vi "Img Crop.vi"(8 "error in (no error)":errorcluster, 10 "Rectangle":T1, 11 "Image Src":T2) -> (0 "error out":errorcluster, 3 "Image Out":T2)   [LabVIEW 2018, in "Image Process.lvclass"]
uses:
  Image Process.lvclass
  <vilib>/vision/Image Controls.llb/IMAQ Image.ctl
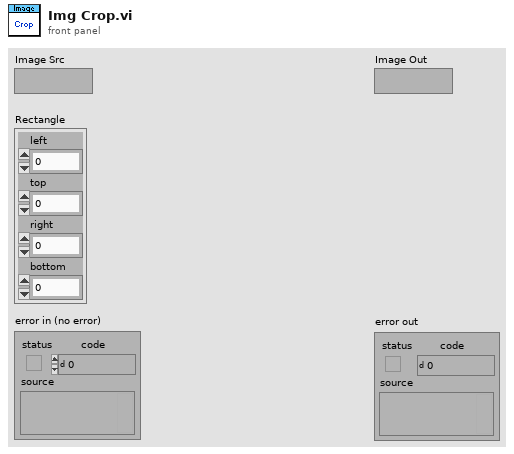
[diagram p1: front panel]
types:
  T1 = cluster{"left":i16, "top":i16, "right":i16, "bottom":i16}
  T2 = typedef "IMAQ Image.ctl" = refnum<image>
  T3 = cluster{"ID":enum32{"External", "Internal"}, "Type":u32, "Coordinates":i32[]}
  T4 = cluster{"ID":enum32{"External", "Internal"}, "Type":u32, "Coordinates":i32[]}[]
  T5 = cluster{"Rectangle":i16[], cluster{"ID":enum32{"External", "Internal"}, "Type":u32, "Coordinates":i32[]}[]}
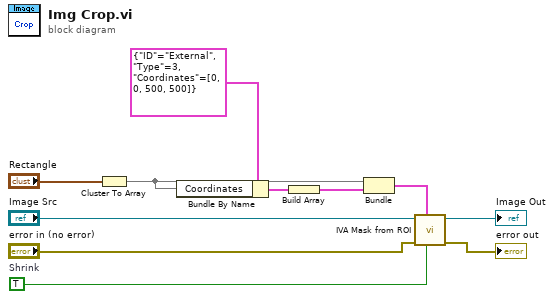
[diagram p0: block diagram]
diagram:
  w11 = TRUE  # Shrink
  n1 = Cluster To Array(cluster="Rectangle") -> (array=w2:i16[])
  n2 = Bundle By Name(cluster=T3 {"ID"=enum."External", "Type"=3, "Coordinates"=[0, 0, 500, 500]}, "Coordinates"=w2) -> (w4:T3)
  n3 = Build Array(w4) -> (w3:T4)
  n4 = Bundle("Rectangle"=w2, w3) -> (w1:T5)  [unwired: 1 in]
  n5 = call <vilib>:"IVA Mask from ROI.vi"("Shrink"=w11, "ROI Descriptor"=w1, "error in (no error)"="error in (no error)", "Image Src"="Image Src") -> ("error out"=→"error out":errorcluster, "Image Out"=→"Image Out":T2)  [unwired: 1 in, 5 out]
